vi "PWM Test.vi"() -> ()   [LabVIEW 2026]
uses:
  <vilib>/eio/EIONode/EIONode.xnode
  <vilib>/rvi/eio/common/nirviEmuTemplateMethod_errors.vi
  Program Files/NI/LVAddons/niidl/1/instr.lib/_niInstr/Basic Elements/v1/FPGA/niInstr Basic Elements v1 FPGA.lvlib
  Program Files/NI/LVAddons/niidl/1/instr.lib/_niInstr/Basic Elements/v1/FPGA/Private/Count Up U16.vi
panel:
  in  "x":u16[](array[numeric])=[0, 0, 0, 0, 0, 0, 0, 0, 0, 0, 0, 0, 0, 0, 0, 0, 0, 0, 0, 0, 0, 0, 0, 0, 0, 0, 0, 0, 0, 0, 0, 0, 0, 0, 0, 0, 0, 0, 0, 0, 0, 0, 0, 0, 0]
  out "Numeric":i32
  in  "Period":u16=100
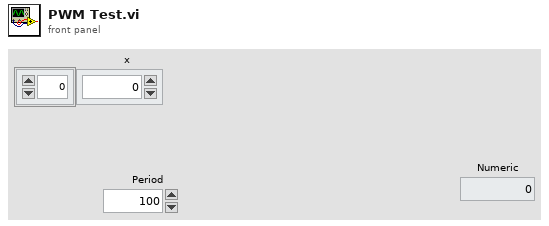
[diagram p1: front panel]
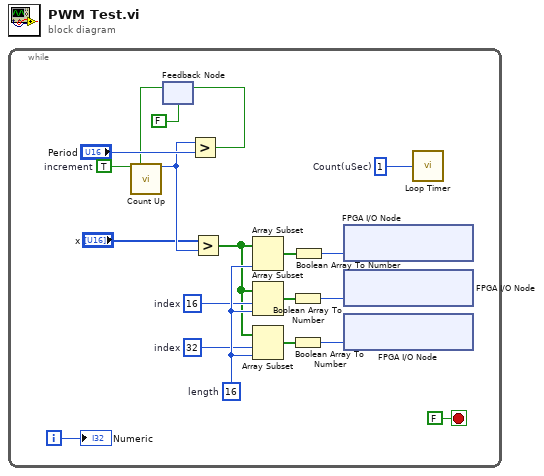
[diagram p0: block diagram]
diagram:
  n1 = while {
    i -> [w17]
    stop <- FALSE stop-if-true
    w5 = 32  # index
    w6 = 16  # index
    w7 = 16  # length
    w15 = u16 1  # Count(uSec)
    w19 = TRUE  # increment
    n2 = feedback #1(FALSE) -> (w14:bool)
    n3 = call-poly "Count Up.vi"("increment"=w19, "reset"=w14) -> ("count out"=w12:u16)  [unwired: 13 in]
    n4 = Greater?(x=w12, y="Period") -> (0:w16:bool)
    n5 = feedback-in #1(w16) -> ()
    n6 = Greater?(x="x", y=w12) -> (0:w3:bool[])
    n7 = Array Subset(array=w3, length=w7) -> (w1:bool[])  [unwired: 1 in]
    n8 = Array Subset(array=w3, index=w6, length=w7) -> (w2:bool[])
    n9 = Array Subset(array=w3, index=w5, length=w7) -> (w4:bool[])
    n10 = Boolean Array To Number(Boolean array=w2) -> (number=w9:u16)
    n11 = Boolean Array To Number(Boolean array=w4) -> (number=w8:u16)
    n12 = Boolean Array To Number(Boolean array=w1) -> (number=w10:u16)
    n13 = xnode "FPGA I/O Node"("Bank-01/DO15:0"=w10) -> ()  [unwired: 1 in, 1 out]
    n14 = xnode "FPGA I/O Node"("Bank-02/DO15:0"=w9) -> ()  [unwired: 1 in, 1 out]
    n15 = xnode "FPGA I/O Node"("Bank-03/DO15:0"=w8) -> ()  [unwired: 1 in, 1 out]
    n16 = call "Loop Timer"("Count(uSec)"=w15) -> ()  [unwired: 1 out]
    "Numeric" <- w17
  }
